vi "SetPathmode.vi"(0 "Pathmode Cluster":T1={"Time [us]"=-inf, "Z Home [nm]"=-2147483600.0, "Edge"=-2147483648} {"Edge" items=["[read only]"=-2147483648, "Raising"=0, "Falling"=1]}, 5 "error in":T3) -> (14 "Output Cluster":T1={"Time [us]"=-inf, "Z Home [nm]"=-2147483600.0, "Edge"=-2147483648} {"Edge" items=["[read only]"=-2147483648, "Raising"=0, "Falling"=1]}, 19 "error out":T3)   [LabVIEW 2016]
doc: "This VI sets all parameters necessary for the path mode and the external trigger. The cluster contains the following:\n- Time (float) [0 to 65535]\n- Edge (integer) [0 -- Raising; 1 -- Falling]\n- Z Home (float) [without restraint]\nBy passing -Inf (float) or -2147483648 (integer) as input values, the corresponding parameter(s) will be read out."
uses:
  Controls/Pathmode_Parameters.ctl
  Controls/Path-Mode-Edge_Selection.ctl
  Controls/Error_Out.ctl
  Files_ASC500/DLL/ASC500_RemoteControlV27.dll
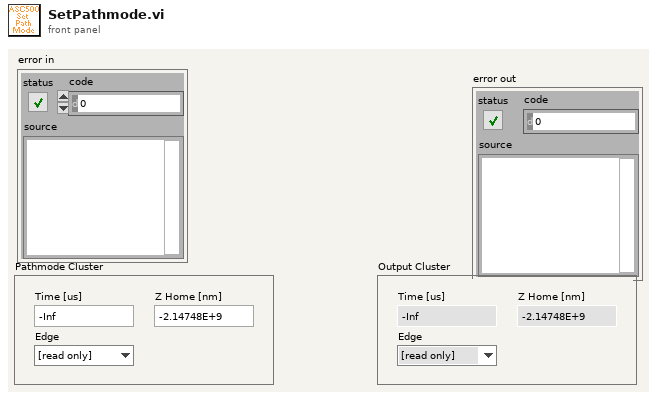
[diagram p1: front panel]
types:
  T1 = typedef "Pathmode_Parameters.ctl" = cluster{"Time [us]":sgl, "Z Home [nm]":sgl, "Edge":T2}
  T2 = typedef "Path-Mode-Edge_Selection.ctl" = i32
  T3 = typedef "Error_Out.ctl" = errorcluster
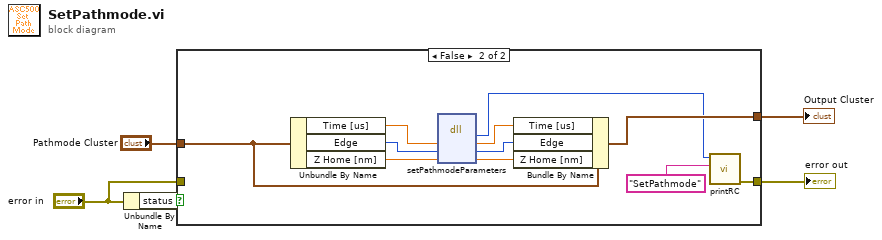
[diagram p0: block diagram]
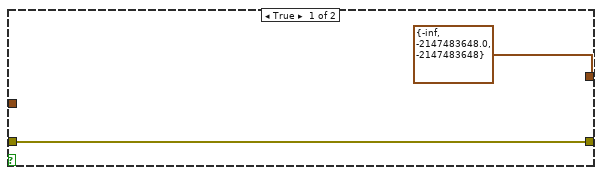
[diagram p2: hidden frame]
diagram:
  n1 = Unbundle By Name("error in") -> ("status"=w5:bool)
  n2 = case shown="False" w5 {
    tunnel: [w6 w9] -> w4
    tunnel: "Pathmode Cluster" -> [_ w13]
    tunnel: [T1 {"Time [us]"=-inf, "Z Home [nm]"=-2147483600.0, "Edge"=-2147483648} ("Pathmode Cluster") w12] -> w2
    tunnel: "error in" -> [w6 _]
    frame True {
    }
    frame False {
      n3 = Unbundle By Name(w13) -> ("Time [us]"=w17:sgl, "Edge"=w18:T2, "Z Home [nm]"=w11:sgl)
      n4 = dll-call lib="G:/SCMOperations/Share/ELE/Produkt Information/ASC500/04 Remote Control/02 development versions/2018Nov06/Files_ASC500/DLL/ASC500_RemoteControlV27.dll" fn="setPathmodeParameters"("Time"=w17, "Edge"=w18, "Z Home"=w11) -> ("return type"=w10:i32, "Time"=w16:sgl, "Edge"=w15:i32, "Z Home"=w14:sgl)  [unwired: 3 in, 2 out]
      n5 = Bundle By Name(cluster=w13, "Time [us]"=w16, "Edge"=w15, "Z Home [nm]"=w14) -> (w12:T1)
      n6 = call "printRC.vi"("additional information"="SetPathmode", "RC"=w10) -> ("error out"=w9:T3)  [unwired: 9 in]
    }
  }
  "error out" <- w4
  "Output Cluster" <- w2
